vi "Parallel PID (DBL).vi"(4 "FeedFwd Value":dbl format="%.2f", 5 "advanced":cluster{"alpha":dbl, "i-zone":dbl}={"alpha"=nan, "i-zone"=nan} {"i-zone" format="%.2f"; "alpha" format="%.2f"}, 6 "reinitialize? (F)":bool, 7 "output range":cluster{"high":dbl, "low":dbl}={"high"=100.0, "low"=-100.0} {"low" format="%.2f"; "high" format="%.2f"}, 8 "dt (s)":dbl=-1.0 format="%.3f", 9 "PID gains":T1={"proportional gain (Kp)"=1.0, "integral time (Ki)"=0.0, "derivative time (Kd)"=0.0} {"derivative time (Kd)" format="%.3f"; "integral time (Ki)" format="%.3f"; "proportional gain (Kp)" format="%.3f"}, 10 "process variable":dbl format="%.2f", 11 "setpoint":dbl format="%.2f") -> (0 "dt out (s)":dbl format="%.3f", 1 "Err/Out Chart":cluster{dbl, dbl}(graph), 2 "SP/PV Chart":cluster{"setpoint":dbl, "process variable":dbl}(graph), 3 "output":dbl format="%.2f")   [LabVIEW 2020]
doc: "Implements a parallel PID controller appropriate for robotics. The PID algorithm features control output range limiting with integrator anti-windup and bumpless controller output for PID gain changes. Include any feedforward amount that should be used to cancel constant forces or improve Velocity control. Advanced params include i-zone to reset integral accumulation on large errors and a derivative smoothing filter."
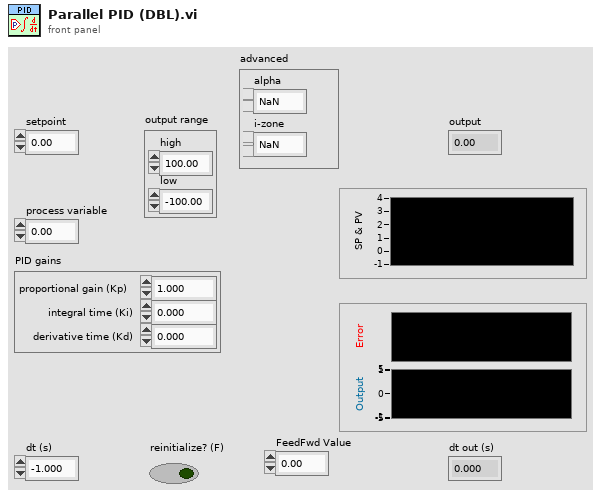
[diagram p1: front panel]
types:
  T1 = cluster{"proportional gain (Kp)":dbl, "integral time (Ki)":dbl, "derivative time (Kd)":dbl}
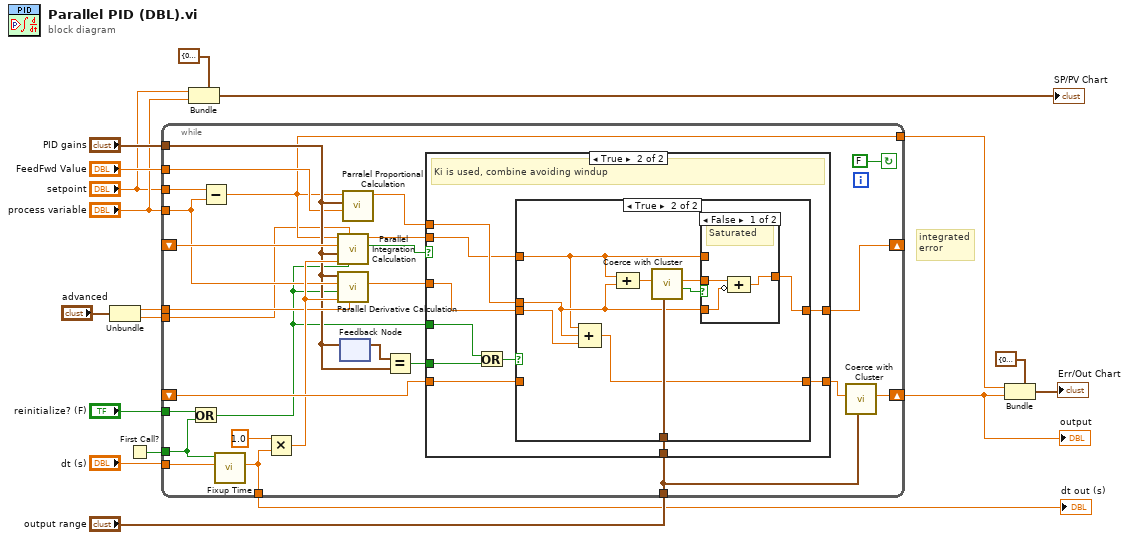
[diagram p0: block diagram]
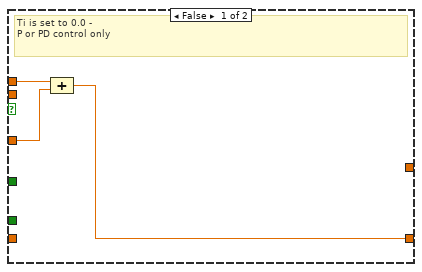
[diagram p2: hidden frame]
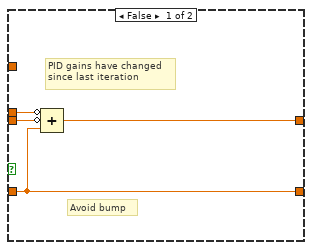
[diagram p3: hidden frame]
diagram:
  # "integrated\nerror"
  n1 = Unbundle("advanced") -> ("alpha"=w2:dbl, "i-zone"=w1:dbl)
  n2 = First Call?() -> (First Call?: T/F=w17:bool)
  n3 = while {
    tunnel: "dt (s)" -> [w41]
    tunnel: "process variable" -> [w30]
    shift-right: [w31] -> w5
    shift-left: _ -> [w44]
    shift-right: [w43] -> _
    shift-left: _ -> [w35]
    tunnel: w17 -> [w28]
    tunnel: "PID gains" -> [w23]
    tunnel: "output range" -> [w33]
    tunnel: [w36] -> w14
    tunnel: "FeedFwd Value" -> [w22]
    tunnel: "setpoint" -> [w29]
    tunnel: "reinitialize? (F)" -> [w27]
    tunnel: [w20] -> w4
    tunnel: w2 -> [w26]
    tunnel: w1 -> [w19]
    stop <- FALSE continue-if-true
    n4 = Or(x=w27, y=w28) -> (x .or. y?=w21:bool)
    n5 = Subtract(x=w29, y=w30) -> (x-y=w20:dbl)
    n6 = call <vilib>:"Fixup Time.vi"("dt (s) in"=w41, "Initialize?:"=w28) -> ("dt (s) out"=w36:dbl)  [unwired: 9 in]
    n7 = Multiply(x=1.0 ("1/60"), y=w36) -> (x*y=w34:dbl)
    n8 = call <vilib>:"Parallel Integration Calculation.vi"("Reinit"=w21, "i-zone"=w19, "dT"=w34, "PID gains"=w23, "Integration Error"=w35, "Curr Error"=w20) -> ("Integral Used"=w38:bool, "Integral Term"=w37:dbl)  [unwired: 4 in]
    n9 = call <vilib>:"Parallel Derivative Calculation.vi"("alpha"=w26, "dt"=w34, "Reinit"=w21, "process variable in"=w30, "PID gains"=w23) -> ("deriv Term"=w45:dbl)  [unwired: 6 in]
    n10 = feedback #1() -> (w25:T1)  [unwired: 1 in]
    n11 = feedback-in #1(w23) -> ()
    n12 = call <vilib>:"Parralel Proportional Calculation.vi"("FeedFwd Amount"=w22, "PID gains"=w23, "Error"=w20) -> ("Proportional Term"=w24:dbl)  [unwired: 8 in]
    n13 = Equal?(x=w25, y=w23) -> (x = y?=w40:bool)
    n14 = case shown="True" w38 {
      tunnel: [_ w55] -> w43
      tunnel: w44 -> [_ w56]
      tunnel: w45 -> [w46 w54]
      tunnel: w21 -> [_ w53]
      tunnel: w40 -> [_ w52]
      tunnel: w33 -> [_ w51]
      tunnel: w37 -> [_ w50]
      tunnel: [w47 w49] -> w32
      tunnel: w24 -> [w48 w58]
      frame False {
        # "Ti is set to 0.0 -\nP or PD control only"
        n15 = Compound Arithmetic op=ADD(w48, w46) -> (w47:dbl)
      }
      frame True {
        # "Ki is used, combine avoiding windup"
        n16 = Or(x=w53, y=w52) -> (x .or. y?=w57:bool)
        n17 = case shown="True" w57 {
          tunnel: w50 -> [_ w63]
          tunnel: w58 -> [w62 w64]
          tunnel: w56 -> [w59 _]
          tunnel: [w60 w71] -> w55
          tunnel: w54 -> [w61 w66]
          tunnel: w51 -> [_ w67]
          tunnel: [w59 w65] -> w49
          frame False {
            # "Avoid bump"
            # "PID gains have changed\nsince last iteration"
            n18 = Compound Arithmetic op=ADD(invert w62, invert w61, w59) -> (w60:dbl)
          }
          frame True {
            n19 = Compound Arithmetic op=ADD(w63, w64, w66) -> (w65:dbl)
            n20 = Compound Arithmetic op=ADD(w63, w64) -> (w68:dbl)
            n21 = call <vilib>:"Coerce with Cluster.vi"("value in"=w68, "output range"=w67) -> ("coerced value"=w69:dbl, "In Range?"=w70:bool)  [unwired: 7 in]
            n22 = case shown="False" w70 {
              tunnel: w63 -> [_ w75]
              tunnel: [w72 w75] -> w71
              tunnel: w69 -> [w74 _]
              tunnel: w64 -> [w73 _]
              frame False {
                # "Saturated"
                n23 = Compound Arithmetic op=ADD(w74, invert w73) -> (w72:dbl)
              }
              frame True {
                # "! Saturated"
              }
            }
          }
        }
      }
    }
    n24 = call <vilib>:"Coerce with Cluster.vi"("value in"=w32, "output range"=w33) -> ("coerced value"=w31:dbl)  [unwired: 7 in, 1 out]
  }
  "output" <- w5
  "dt out (s)" <- w14
  n25 = Bundle(cluster=cluster{"setpoint":dbl, "process variable":dbl} {"setpoint"=0.0, "process variable"=0.0}, "setpoint"="setpoint", "process variable"="process variable") -> (→"SP/PV Chart":cluster{"setpoint":dbl, "process variable":dbl})
  n26 = Bundle(cluster=cluster{"Error":dbl, "Output":dbl} {"Error"=0.0, "Output"=0.0}, "Error"=w4, "Output"=w5) -> (→"Err/Out Chart":cluster{"Error":dbl, "Output":dbl})
